vi "Initialize Do.vi"(8 "error in (no error)":errorcluster, 11 "Instrument in":refnum<class "DMM.NI.lvclass">) -> (0 "error out":errorcluster, 3 "Instrument out":refnum<class "DMM.NI.lvclass">)   [LabVIEW 2020, in "NI DMM Driver.lvlib" / "DMM.NI.lvclass"]
doc: "Initialize the Instrument.\n\nInitialize the NI DMM with the contained Alias."
uses:
  DMM.NI.lvclass
  DMM.NI.lvclass/DMM.NI.ctl
  PPL/HDH.Driver.DMM.lvlibp/DMM Driver.lvclass
  PPL/HDH.Actor Framework.Core.Instrument Driver.lvlibp/Instrument Driver/Instrument Driver.lvclass
  C:/Current Projects/WS/PPL/HDH.Actor Framework.Core.Instrument Driver.lvlibp/Instrument Driver/Instrument Driver.lvclass
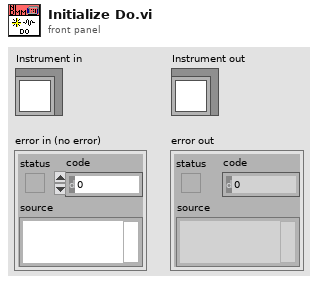
[diagram p1: front panel]
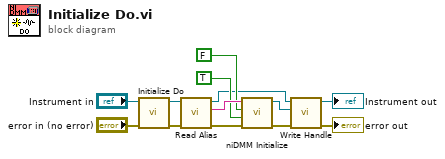
[diagram p0: block diagram]
diagram:
  n1 = call-parent "Initialize Do.vi"("error in (no error)"="error in (no error)", "Instrument in"="Instrument in") -> ("error out"=w7:errorcluster, "Instrument out"=w11:refnum<class "DMM.NI.lvclass">)  [unwired: 8 in]
  n2 = call "Read Alias.vi"("error in (no error)"=w7, "Instrument in"=w11) -> ("error out"=w6:errorcluster, "Alias"=w10:string, "Instrument out"=w5:refnum<class "DMM.NI.lvclass">)  [unwired: 7 in]
  n3 = call <instrlib>:"niDMM Initialize.vi"("error in (no error)"=w6, "Reset"=TRUE, "ID Query"=FALSE, "Instrument Descriptor"=w10) -> ("error out"=w2:errorcluster, "instrument handle out"=w4:refnum<k15>)  [unwired: 6 in]
  n4 = call "Write Handle.vi"("error in (no error)"=w2, "NI DMM"=w4, "NI DMM Driver in"=w5) -> ("error out"=→"error out":errorcluster, "NI DMM Driver out"=→"Instrument out":refnum<class "DMM.NI.lvclass">)  [unwired: 7 in]
